vi "Configure Average.vi"(7 "Average On":bool, 8 "error in (no error)":errorcluster, 10 "Number of Averages":i32, 11 "VNA-ZNB in":refnum<class "VNA-ZNB.lvclass">) -> (0 "error out":errorcluster, 3 "VNA-ZNB out":refnum<class "VNA-ZNB.lvclass">)   [LabVIEW 2020, in "VNA-ZNB.lvclass"]
doc: "Configures the average to use for the sweep"
uses:
  VNA-ZNB.lvclass
  C:/Sandbox/RF Bench/Source Code/WiSpry Test Framework/Instruments/Instrument.lvclass
  C:/Sandbox/RF Bench/Source Code/WiSpry Test Framework/Instruments/Vector Network Analyzer/Vector Network Analyzer.lvclass
  Instrument.lvclass/Instrument.ctl
  Vector Network Analyzer.lvclass/Vector Network Analyzer.ctl
  Instrument.lvclass
  Vector Network Analyzer.lvclass
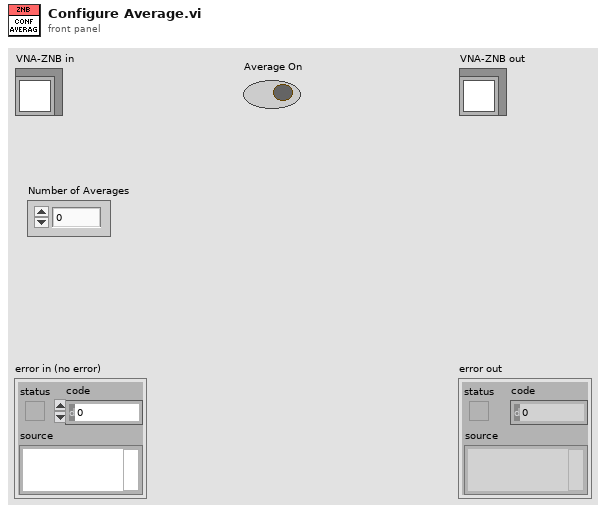
[diagram p1: front panel]
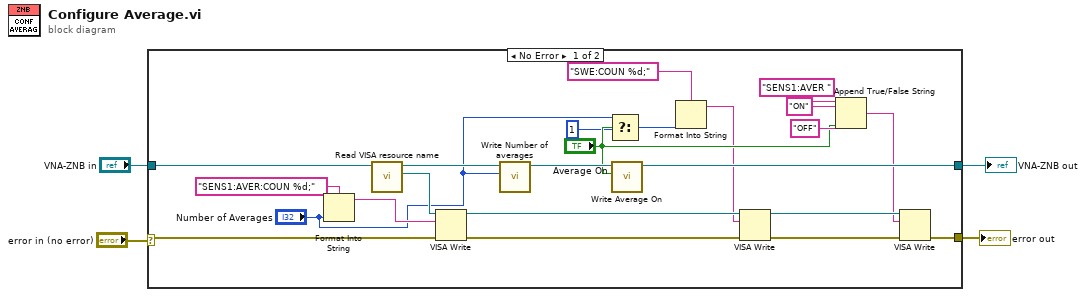
[diagram p0: block diagram]
diagram:
  n1 = case shown="No Error" "error in (no error)" {
    selector: "error in (no error)" -> [w25 w28]
    tunnel: "VNA-ZNB in" -> [w26 w29]
    tunnel: [w18 w29] -> w1
    tunnel: [w11 w28] -> w2
    frame No Error {
      n2 = Format Into String(format string="SENS1:AVER:COUN %d;", "Number of Averages") -> (resulting string=w23:string)  [unwired: 2 in, 1 out]
      n3 = call "Read VISA resource name.vi"("Instrument in"=w26) -> ("VISA resource name"=w24:refnum<visa-resource-name>, "Instrument out"=w20:refnum<class "VNA-ZNB.lvclass">)  [unwired: 9 in]
      n4 = VISA Write(VISA resource name=w24, write buffer=w23, error in (no error)=w25) -> (VISA resource name out=w9:refnum<visa-resource-name>, error out=w10:errorcluster)  [unwired: 1 out]
      n5 = call "Write Number of averages.vi"("Number of averages"="Number of Averages", "Vector Network Analyzer in"=w20) -> ("Vector Network Analyzer out"=w19:refnum<class "VNA-ZNB.lvclass">)  [unwired: 9 in]
      n6 = Select(t="Number of Averages", s="Average On", f=1) -> (s? t:f=w12:i32)
      n7 = call "Write Average On.vi"("Average On"="Average On", "Vector Network Analyzer in"=w19) -> ("Vector Network Analyzer out"=w18:refnum<class "VNA-ZNB.lvclass">)  [unwired: 9 in]
      n8 = Format Into String(format string="SWE:COUN %d;", w12) -> (resulting string=w8:string)  [unwired: 2 in, 1 out]
      n9 = VISA Write(VISA resource name=w9, write buffer=w8, error in (no error)=w10) -> (VISA resource name out=w6:refnum<visa-resource-name>, error out=w7:errorcluster)  [unwired: 1 out]
      n10 = Append True/False String(1:"Average On", 2:"OFF" ("false string"), 3:"ON" ("true string"), 4:"SENS1:AVER " ("string (\"\")")) -> (0:w5:string)
      n11 = VISA Write(VISA resource name=w6, write buffer=w5, error in (no error)=w7) -> (error out=w11:errorcluster)  [unwired: 2 out]
    }
    frame Error {
    }
  }
  "error out" <- w2
  "VNA-ZNB out" <- w1
